vi "SENS_BAND_BWID_RES.vi"(0 "VISA IN":refnum<visa-resource-name>, 5 "error in":errorcluster, 7 "Channel":i32, 9 "Resolution":dbl) -> (14 "VISA Out":refnum<visa-resource-name>, 19 "error out":errorcluster)   [LabVIEW 2018, in "PNA-X.lvlib"]
doc: "SENSe<cnum>:BANDwidth | BWIDth[:RESolution] <num> \n(Read-Write) Sets the bandwidth of the digital IF filter to be used in the measurement. (Use either \nSense:Bandwidth or Sense:Bwidth) \nParameters \n<cnum> Any existing channel number. If unspecified, value is set to 1 \n<num> IF Bandwidth in Hz. The list of valid IF Bandwidths is different depending on \nthe PNA model. (Click to see the lists.) If an invalid number is specified, the \nanalyzer will round up to the closest valid number. \nExamples SENS:BWID 1KHZ \nsense2:bandwidth:resolution 1000 \nQuery Syntax SENSe<cnum>:BANDwidth | BWIDth[:RESolution]? \nReturn Type Numeric \nDefault See Preset IFBW for your PNA model."
uses:
  PNA-X.lvlib
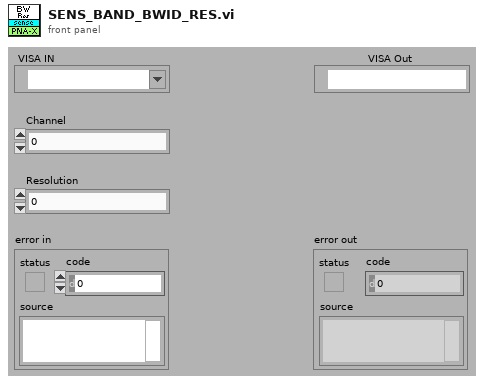
[diagram p1: front panel]
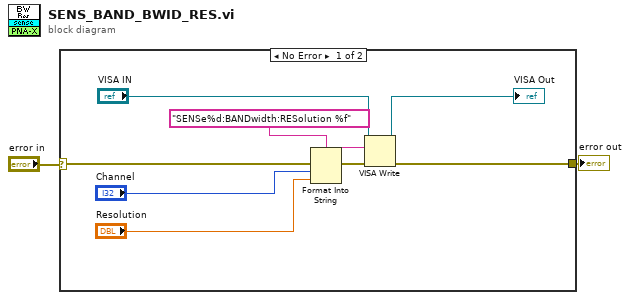
[diagram p0: block diagram]
diagram:
  n1 = case shown="No Error" "error in" {
    selector: "error in" -> [w11 w12]
    tunnel: [w6 w12] -> w1
    frame No Error {
      n2 = Format Into String(format string="SENSe%d:BANDwidth:RESolution %f" ("Cmdline"), error in=w11, "Channel", "Resolution") -> (resulting string=w9:string, error out=w10:errorcluster)  [unwired: 1 in]
      n3 = VISA Write(VISA resource name="VISA IN", write buffer=w9, error in (no error)=w10) -> (VISA resource name out=→"VISA Out":refnum<visa-resource-name>, error out=w6:errorcluster)  [unwired: 1 out]
    }
    frame Error {
    }
  }
  "error out" <- w1
